vi "Get 32-bit Image Subset.vi"(4 "subset rect":T1, 6 "image data":T2) -> (0 "true subset rect":T1, 2 "image subset":T2)   [LabVIEW 2021, in "Picture2D.lvlib"]
doc: "<p>Returns a subset of a source image instead of the entire image. Use the <a href=\"nihelplauncher://docs/csh?context=lvcore_lvpict_picture_to_pixmap\">Picture to Pixmap</a> VI to convert a picture to a cluster you can wire to <strong>image data</strong>.</p>"
uses:
  Picture2D/Picture2D.lvlib
  <vilib>/picture/picture.llb/imagedata.ctl
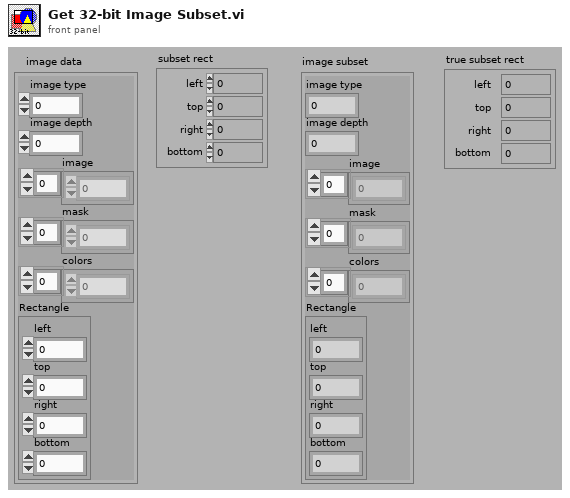
[diagram p1: front panel]
types:
  T1 = cluster{"left":i16, "top":i16, "right":i16, "bottom":i16}
  T2 = typedef "imagedata.ctl" = cluster{"image type":i32, "image depth":i32, "image":u8[], "mask":u8[], "colors":u32[], "Rectangle":cluster{"left":i16, "top":i16, "right":i16, "bottom":i16}}
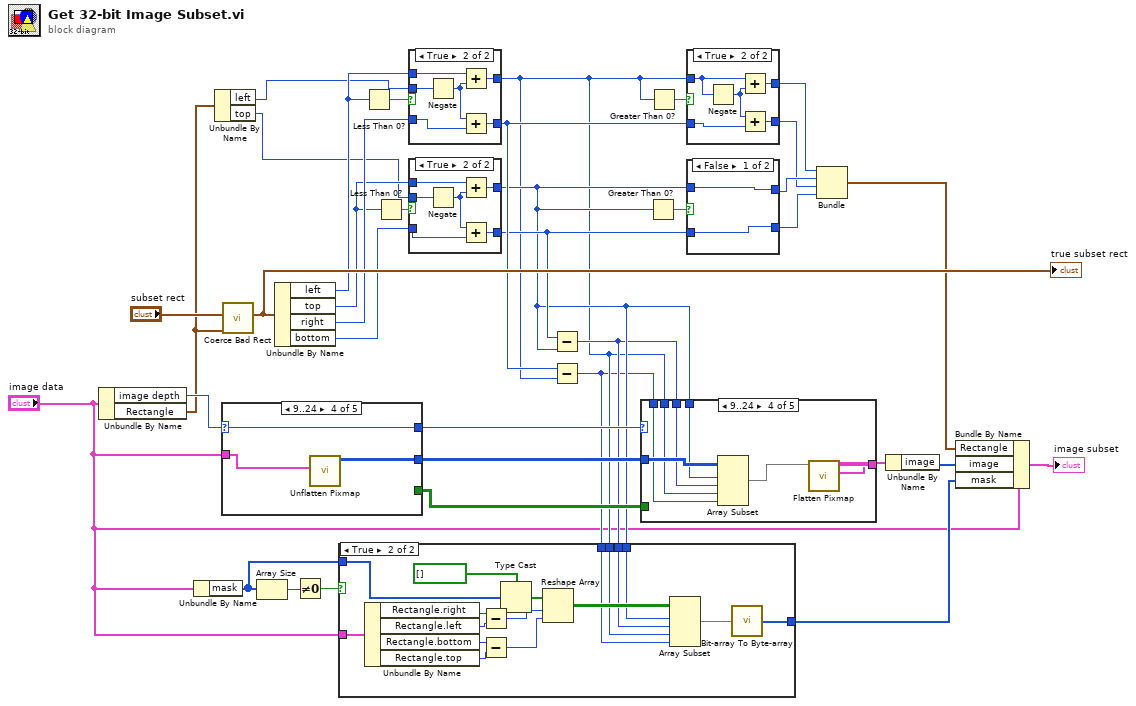
[diagram p0: block diagram]
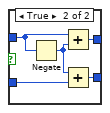
[diagram p3: hidden frame]
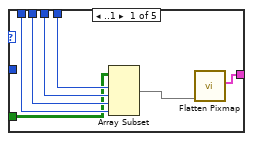
[diagram p7: hidden frame]
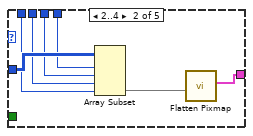
[diagram p8: hidden frame]
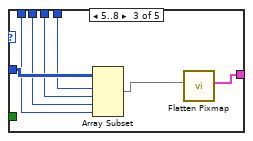
[diagram p9: hidden frame]
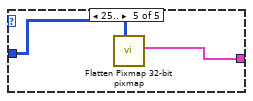
[diagram p10: hidden frame]
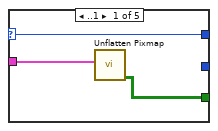
[diagram p11: hidden frame]
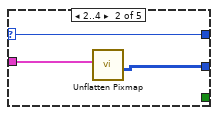
[diagram p12: hidden frame]
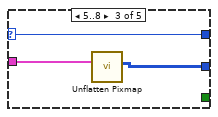
[diagram p13: hidden frame]
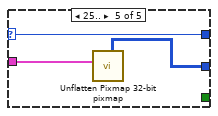
[diagram p14: hidden frame]
diagram:
  n1 = Unbundle By Name("image data") -> ("image depth"=w34:i32, "Rectangle"=w14:T1)
  n2 = Unbundle By Name("image data") -> ("mask"=w2:u8[])
  n3 = Unbundle By Name(w14) -> ("left"=w13:i16, "top"=w12:i16)
  n4 = case shown="9..24" w34 {
    selector: w34 -> [w39 w42 w45 w46 w49]
    tunnel: [_ w41 w44 w48 w50] -> w35
    tunnel: [w38 _ _ _ _] -> w36
    tunnel: [w39 w42 w45 w46 w49] -> w31
    tunnel: "image data" -> [w37 w40 w43 w47 w51]
    frame ..1 {
      n5 = call <vilib>:"Unflatten Pixmap.vi"("image data"=w37) -> ("1-bit pixmap"=w38:bool[][])  [unwired: 4 in, 6 out]
    }
    frame 2..4 {
      n6 = call <vilib>:"Unflatten Pixmap.vi"("image data"=w40) -> ("4-bit pixmap"=w41:u8[][])  [unwired: 4 in, 6 out]
    }
    frame 5..8 {
      n7 = call <vilib>:"Unflatten Pixmap.vi"("image data"=w43) -> ("8-bit pixmap"=w44:u8[][])  [unwired: 4 in, 6 out]
    }
    frame 9..24 {
      n8 = call <vilib>:"Unflatten Pixmap.vi"("image data"=w47) -> ("24-bit pixmap"=w48:u32[][])  [unwired: 4 in, 6 out]
    }
    frame 25.. {
      n9 = call "Unflatten Pixmap 32-bit pixmap.vi"("image data"=w51) -> ("32-bit pixmap"=w50:u32[][])  [unwired: 3 in, 7 out]
    }
  }
  n10 = call <vilib>:"Coerce Bad Rect.vi"("image rect"=w14, "subset rect"="subset rect") -> ("Rectangle"=w29:T1)  [unwired: 9 in]
  "true subset rect" <- w29
  n11 = Array Size(array=w2) -> (size(s)=w4:i32)
  n12 = Unbundle By Name(w29) -> ("left"=w26:i16, "top"=w24:i16, "right"=w27:i16, "bottom"=w23:i16)
  n13 = Not Equal To 0?(x=w4) -> (x != 0?=w3:bool)
  n14 = Less Than 0?(x=w26) -> (x < 0?=w28:bool)
  n15 = Less Than 0?(x=w24) -> (x < 0?=w25:bool)
  n16 = case shown="True" w28 {
    tunnel: w26 -> [w53 w55]
    tunnel: w27 -> [w52 w56]
    tunnel: [w53 w59] -> w9
    tunnel: [w52 w57] -> w21
    tunnel: w13 -> [_ w54]
    frame False {
    }
    frame True {
      n17 = Negate(x=w54) -> (-x=w58:i16)
      n18 = Add(x=w55, y=w58) -> (x+y=w59:i16)
      n19 = Add(x=w58, y=w56) -> (x+y=w57:i16)
    }
  }
  n20 = case shown="True" w25 {
    tunnel: w24 -> [w61 w63]
    tunnel: w23 -> [w60 w65]
    tunnel: [w61 w67] -> w11
    tunnel: [w60 w64] -> w19
    tunnel: w12 -> [_ w62]
    frame False {
    }
    frame True {
      n21 = Negate(x=w62) -> (-x=w66:i16)
      n22 = Add(x=w63, y=w66) -> (x+y=w67:i16)
      n23 = Add(x=w66, y=w65) -> (x+y=w64:i16)
    }
  }
  n24 = Subtract(x=w19, y=w11) -> (x-y=w10:i16)
  n25 = Subtract(x=w21, y=w9) -> (x-y=w8:i16)
  n26 = case shown="True" w3 {
    tunnel: w11 -> [_ w76]
    tunnel: w10 -> [_ w75]
    tunnel: w9 -> [_ w74]
    tunnel: w8 -> [_ w73]
    tunnel: [w68 w71] -> w7
    tunnel: "image data" -> [_ w70]
    tunnel: w2 -> [w68 w69]
    frame False {
    }
    frame True {
      n27 = Unbundle By Name(w70) -> ("Rectangle.right"=w83:i16, "Rectangle.left"=w82:i16, "Rectangle.bottom"=w80:i16, "Rectangle.top"=w79:i16)
      n28 = Subtract(x=w83, y=w82) -> (x-y=w81:i16)
      n29 = Subtract(x=w80, y=w79) -> (x-y=w78:i16)
      n30 = Type Cast(type=bool[] [], x=w69) -> (*(type *) &x=w84:bool[])
      n31 = Reshape Array(w84, w81, w78) -> (w77:bool[][])
      n32 = Array Subset(array=w77, index (row)=w76, length (row)=w75, index (col)=w74, length (col)=w73) -> (w72:bool[][])
      n33 = call <vilib>:"Bit-array To Byte-array.vi"("bit array"=w72) -> ("byte array"=w71:u8[])
    }
  }
  n34 = case shown="9..24" w31 {
    tunnel: w35 -> [_ w98 w106 w113 w115]
    tunnel: w36 -> [w86 _ _ _ _]
    tunnel: w11 -> [w92 w96 w103 w110 _]
    tunnel: w10 -> [w91 w94 w101 w108 _]
    tunnel: w9 -> [w90 w95 w102 w109 _]
    tunnel: w8 -> [w89 w93 w100 w107 _]
    tunnel: [w87 w97 w104 w111 w114] -> w32
    frame ..1 {
      n35 = Array Subset(array=w86, index (row)=w92, length (row)=w91, index (col)=w90, length (col)=w89) -> (w88:bool[][])
      n36 = call <vilib>:"Flatten Pixmap.vi"("1-bit pixmap"=w88) -> ("image data"=w87:T2)  [unwired: 10 in]
    }
    frame 2..4 {
      n37 = Array Subset(array=w98, index (row)=w96, length (row)=w94, index (col)=w95, length (col)=w93) -> (w99:u32[][])
      n38 = call <vilib>:"Flatten Pixmap.vi"("4-bit pixmap"=w99) -> ("image data"=w97:T2)  [unwired: 10 in]
    }
    frame 5..8 {
      n39 = Array Subset(array=w106, index (row)=w103, length (row)=w101, index (col)=w102, length (col)=w100) -> (w105:u32[][])
      n40 = call <vilib>:"Flatten Pixmap.vi"("8-bit pixmap"=w105) -> ("image data"=w104:T2)  [unwired: 10 in]
    }
    frame 9..24 {
      n41 = Array Subset(array=w113, index (row)=w110, length (row)=w108, index (col)=w109, length (col)=w107) -> (w112:u32[][])
      n42 = call <vilib>:"Flatten Pixmap.vi"("24-bit pixmap"=w112) -> ("image data"=w111:T2)  [unwired: 10 in]
    }
    frame 25.. {
      n43 = call "Flatten Pixmap 32-bit pixmap.vi"("32-bit pixmap"=w115) -> ("image data"=w114:T2)  [unwired: 10 in]
    }
  }
  n44 = Greater Than 0?(x=w11) -> (x > 0?=w20:bool)
  n45 = Greater Than 0?(x=w9) -> (x > 0?=w22:bool)
  n46 = case shown="True" w22 {
    tunnel: w9 -> [w117 w122]
    tunnel: w21 -> [w116 w120]
    tunnel: [w117 w119] -> w18
    tunnel: [w116 w118] -> w16
    frame False {
    }
    frame True {
      n47 = Negate(x=w122) -> (-x=w121:i16)
      n48 = Add(x=w122, y=w121) -> (x+y=w119:i16)
      n49 = Add(x=w121, y=w120) -> (x+y=w118:i16)
    }
  }
  n50 = case shown="False" w20 {
    tunnel: w11 -> [w124 w128]
    tunnel: w19 -> [w123 w127]
    tunnel: [w124 w126] -> w17
    tunnel: [w123 w125] -> w15
    frame False {
    }
    frame True {
      n51 = Negate(x=w128) -> (-x=w129:i16)
      n52 = Add(x=w128, y=w129) -> (x+y=w126:i16)
      n53 = Add(x=w129, y=w127) -> (x+y=w125:i16)
    }
  }
  n54 = Bundle("left"=w18, "top"=w17, "right"=w16, "bottom"=w15) -> (w6:T1)  [unwired: 1 in]
  n55 = Unbundle By Name(w32) -> ("image"=w5:u8[])
  n56 = Bundle By Name(cluster="image data", "Rectangle"=w6, "image"=w5, "mask"=w7) -> (→"image subset":T2)
